vi "ADC_ForceTrig.vi"(8 "error in (no error)":errorcluster) -> (0 "error out":errorcluster, 3 "function return":i16)   [LabVIEW 2013, in "MeasurmentRoutines.lvlib"]
doc: "Description: This routine forces a trigger when the input signal will not meet the trigger specifications. This allows to do a measurement and see the signal.\nInput: -\nOutput: Return value E_NOT_INITIALIZED | E_NO_ERRORS | E_NO_HARDWARE\n\n\nFunction prototype: word ADC_ForceTrig( void )\n\n\n\nshort int ADC_ForceTrig ( void );"
uses:
  MeasurmentRoutines.lvlib
  hs3.dll
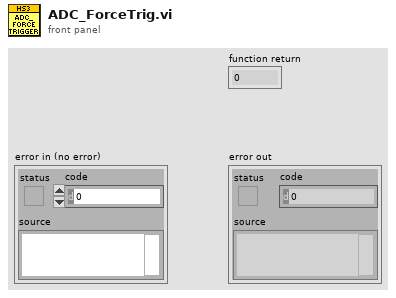
[diagram p1: front panel]
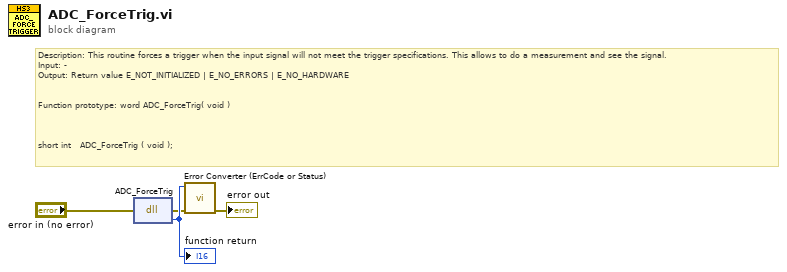
[diagram p0: block diagram]
diagram:
  # "Description: This routine forces a trigger when the input signal will not meet the trigger specifications. This allows to do a measurement and see the signal.\nInput: -\nOutput: Return value E_NOT_INITIALIZED | E_NO_ERRORS | E_NO_HARDWARE\n\n\nFunction prototype: word ADC_ForceTrig( void )\n\n\n\nshort int \t\tADC_ForceTrig\t( void );"
  n1 = dll-call lib="C:/Documents and Settings/admin/Pulpit/HS3 LabViewLib/HS3_WRAPPER/hs3.*" fn="ADC_ForceTrig"(error in="error in (no error)") -> (error out=w2:errorcluster, w4:i16)  [unwired: 2 in, 1 out]
  "function return" <- w4
  n2 = call "Error Converter (ErrCode or Status).vi"("error in (no error)"=w2, "error code"=w4) -> ("error out"=→"error out":errorcluster)  [unwired: 9 in]
